vi "Predefined_SuperUser.vi"() -> (3 "SuperUsers":T1[](array[typedef]))   [LabVIEW 2020]
uses:
  Typedef/User-Info.ctl
  Typedef/User-Role.ctl
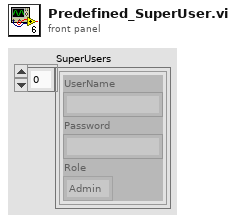
[diagram p1: front panel]
types:
  T1 = typedef "User-Info.ctl" = cluster{"UserName":string, "Password":string, "Role":T2}
  T2 = typedef "User-Role.ctl" = enum16{"Admin", "Engineer", "Operator"}
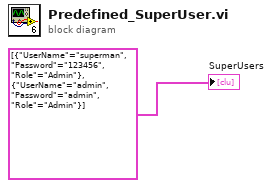
[diagram p0: block diagram]
diagram:
  "SuperUsers" <- T1[] [{"UserName"="superman", "Password"="123456", "Role"=enum."Admin"}, {"UserName"="admin", "Password"="admin", "Role"=enum."Admin"}] ("Array")
